vi "Connect4.vi"() -> ()   [LabVIEW 2014]
panel:
  out "Clicked Index":i32[](array[numeric])
  out "Array 2":enum16{"Blank", "Player 1", "Player 2"}[][](array[ring])
  in  "stop":bool
  out "Array":bool[][](array[boolean])
  in  "Player 2 Color":u32(colorbox)
  in  "Player 1 Color":u32(colorbox)
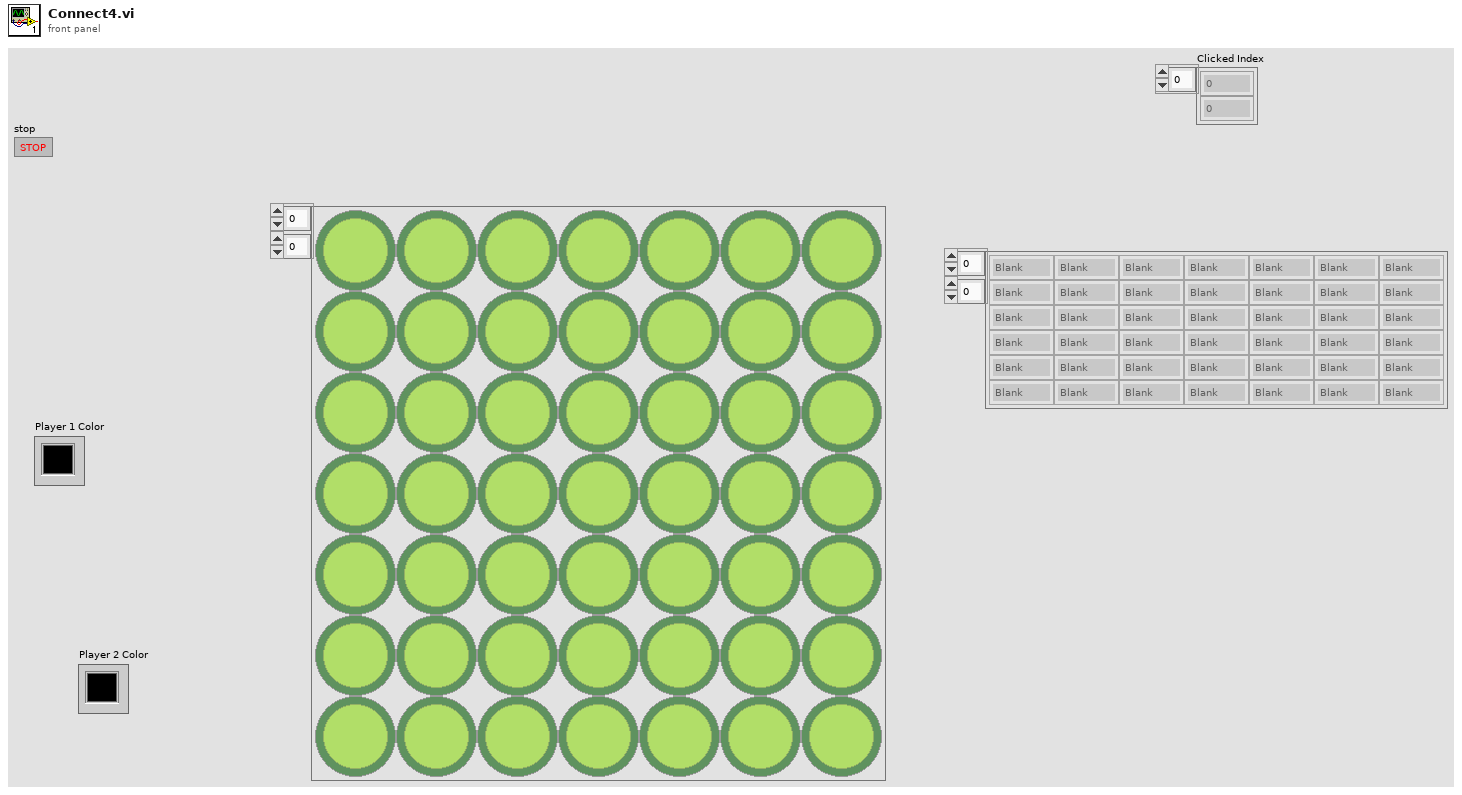
[diagram p1: front panel]
types:
  T1 = cluster{"Player 2 Color ":u32, "Player 2 Color ":u32}
  T2 = cluster{"Player 2 Color ":u32, "Player 2 Color ":u32}[]
  T3 = cluster{"Player 1 Color":u32, "Player 1 Color":u32}
  T4 = cluster{"Player 1 Color":u32, "Player 1 Color":u32}[]
  T5 = typedef "LVPoint32TypeDef.ctl" = cluster{"Horizontal":i32, "Vertical":i32}
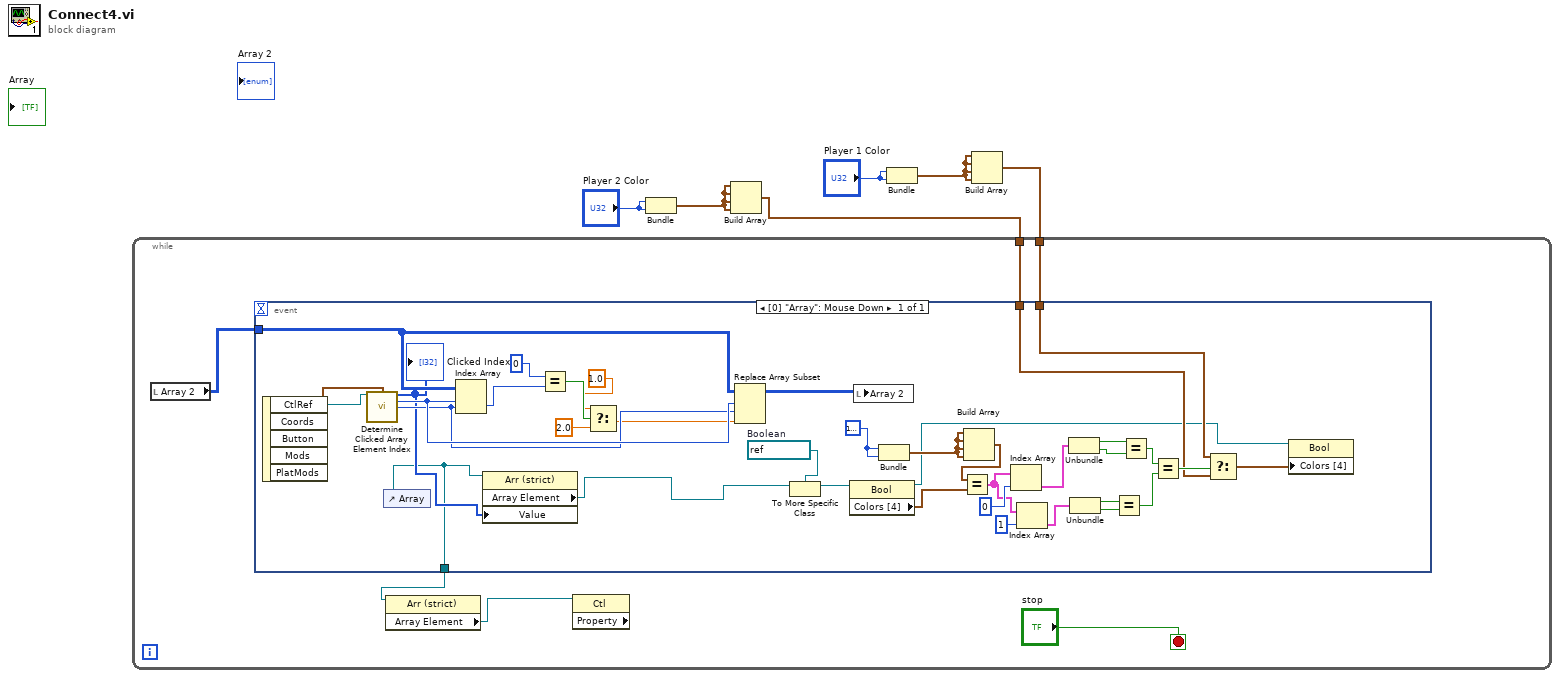
[diagram p0: block diagram]
diagram:
  n1 = Bundle("Player 2 Color"="Player 2 Color", "Player 2 Color"="Player 2 Color") -> (w3:T1)  [unwired: 1 in]
  n2 = Build Array(w3, w3, w3, w3) -> (w1:T2)
  n3 = Bundle("Player 1 Color"="Player 1 Color", "Player 1 Color"="Player 1 Color") -> (w5:T3)  [unwired: 1 in]
  n4 = Build Array(w5, w5, w5, w5) -> (w2:T4)
  n5 = while {
    tunnel: w2 -> [w10]
    tunnel: w1 -> [w9]
    stop <- "stop" stop-if-true
    n6 = local read "Array 2"() -> (w11:enum16{"Blank", "Player 1", "Player 2"}[][])
    n7 = event shown="[0] \"Array\": Mouse Down" {
      selector: _ -> [_]
      dyn-events: _ -> [_]
      timeout: _ -> [_]
      tunnel: w11 -> [w42]
      tunnel: w10 -> [w21]
      tunnel: w9 -> [w20]
      tunnel: [w13] -> w7
      event "Array": Mouse Down {
        w35 = u32 16777222
        w37 = refnum<vi> refnum  # Boolean
        n8 = event-data() -> ("CtlRef"=w48:refnum<vi>, "Coords"=w49:T5)  [unwired: 1 in, 3 out]
        n9 = call "Determine Clicked Array Element Index.vi"("reference"=w48, "Coords of Click"=w49) -> ("Clicked Index"=w14:i32[], "Clicked Row"=w41:i32, "Clicked Col"=w40:i32)  [unwired: 8 in, 3 out]
        "Clicked Index" <- w14
        n10 = control-ref of="Array"() -> (w13:refnum<vi>)
        n11 = Index Array(array=w42, index (row)=w41, index (col)=w40) -> (element=w47:enum16{"Blank", "Player 1", "Player 2"})
        n12 = property class="Arr (strict)"(reference=w13, "Value"=w14) -> ("Array Element"=w15:refnum<vi>)  [unwired: 1 in, 2 out]
        n13 = Equal?(x=0, y=w47) -> (x = y?=w46:bool)
        n14 = Select(t=1.0 ("f"), s=w46, f=2.0) -> (s? t:f=w39:dbl)
        n15 = Replace Array Subset(array=w42, new element=w39, index (row)=w41, index (col)=w40) -> (w38:enum16{"Blank", "Player 1", "Player 2"}[][])
        n16 = To More Specific Class(target class=w37, reference=w15) -> (specific class reference=w36:refnum<vi>)  [unwired: 1 in, 1 out]
        n17 = property class="Bool"(reference=w36) -> (reference out=w16:refnum<vi>, "Colors [4]"=w34:cluster{u32, u32}[])  [unwired: 1 in, 1 out]
        n18 = local write "Array 2"(w38) -> ()
        n19 = Bundle(w35, w35) -> (w17:cluster{u32, u32})  [unwired: 1 in]
        n20 = Build Array(w17, w17, w17, w17) -> (w18:cluster{u32, u32}[])
        n21 = Equal?(x=w18, y=w34) -> (x = y?=w30:cluster{bool, bool}[])
        n22 = Index Array(array=w30, index=0) -> (element=w32:cluster{bool, bool})
        n23 = Index Array(array=w30, index=1) -> (element=w29:cluster{bool, bool})
        n24 = Unbundle(w32) -> (w28:bool, w27:bool)
        n25 = Unbundle(w29) -> (w26:bool, w25:bool)
        n26 = Equal?(x=w26, y=w25) -> (x = y?=w23:bool)
        n27 = Equal?(x=w28, y=w27) -> (x = y?=w24:bool)
        n28 = Equal?(x=w24, y=w23) -> (x = y?=w22:bool)
        n29 = Select(t=w21, s=w22, f=w20) -> (s? t:f=w19:T2)
        n30 = property class="Bool"(reference=w16, "Colors [4]"=w19) -> ()  [unwired: 1 in, 2 out]
      }
    }
    n31 = property class="Arr (strict)"(reference=w7) -> ("Array Element"=w8:refnum<vi>)  [unwired: 1 in, 2 out]
    n32 = property class="Ctl" props=[](reference=w8) -> ()  [unwired: 1 in, 3 out]
  }
